vi "stop_py.vi"(4 "error in":errorcluster, 6 "Python session":refnum<k35>) -> (0 "error out":errorcluster)   [LabVIEW 2018]
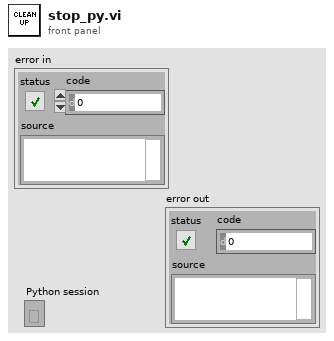
[diagram p1: front panel]
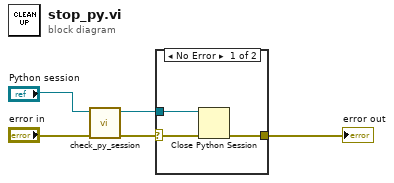
[diagram p0: block diagram]
diagram:
  n1 = call "check_py_session.vi"("error in"="error in", "Python session in"="Python session") -> ("error out"=w3:errorcluster, "Python session out"=w1:refnum<k35>)  [unwired: 3 in, 1 out]
  n2 = case shown="No Error" w3 {
    selector: w3 -> [w8 w9]
    tunnel: [w7 w9] -> w5
    tunnel: w1 -> [w6 _]
    frame No Error {
      n3 = Close Python Session(session in=w6, error in=w8) -> (11:w7:errorcluster)
    }
    frame Error {
    }
  }
  "error out" <- w5
